vi "OpenTemplateVIs.vi"   [LabVIEW 2020]
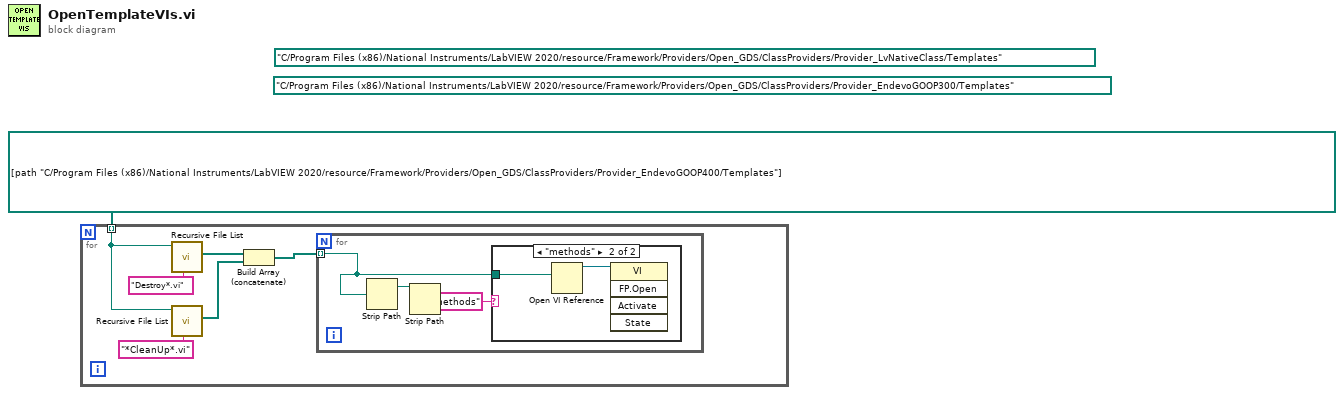
[diagram p0: block diagram]
diagram:
  (unwired) path "C:/Program Files (x86)/National Instruments/LabVIEW 2020/resource/Framework/Providers/Open_GDS/ClassProviders/Provider_EndevoGOOP300/Templates" ("Folder to Search")
  (unwired) path "C:/Program Files (x86)/National Instruments/LabVIEW 2020/resource/Framework/Providers/Open_GDS/ClassProviders/Provider_LvNativeClass/Templates" ("Folder to Search")
  n1 = for {
    tunnel: path[] [path "C:/Program Files (x86)/National Instruments/LabVIEW 2020/resource/Framework/Providers/Open_GDS/ClassProviders/Provider_EndevoGOOP400/Templates"] ("Folders to Search") -> [w4] mode=indexing
    n2 = call <vilib>:"Recursive File List.vi"("pattern"="Destroy*.vi", "Folder Path"=w4) -> ("All Files in Dir"=w6:path[])  [unwired: 5 in, 4 out]
    n3 = call <vilib>:"Recursive File List.vi"("pattern"="*CleanUp*.vi", "Folder Path"=w4) -> ("All Files in Dir"=w2:path[])  [unwired: 5 in, 4 out]
    n4 = Build Array (concatenate)(w6, w2) -> (w3:path[])
    n5 = for {
      tunnel: w3 -> [w10] mode=indexing
      n6 = Strip Path(path=w10) -> (stripped path=w9:path)  [unwired: 1 out]
      n7 = Strip Path(path=w9) -> ()  [unwired: 2 out]
      n8 = case shown="\"methods\"" "methods" {
        tunnel: w10 -> [_ w11]
        frame "False", Default {
        }
        frame "methods" {
          n9 = Open VI Reference(vi path=w11) -> (vi reference=w12:refnum<vi>)  [unwired: 5 in, 1 out]
          n10 = invoke class="VI" method="FP.Open"(reference=w12) -> ()  [unwired: 4 in, 5 out]
        }
      }
    }
  }
